vi "Analog Input.vi"() -> ()   [LabVIEW 2016]
doc: "This VI will read single point values from 4 channels of a R Series board at a specified rate."
uses:
  <vilib>/rvi/Emulation/niFpgaGetClockAttributes.vi
  <vilib>/rvi/Emulation/niFpgaSctlEmulationGetInTimedLoop.vi
  <vilib>/rvi/Emulation/niFpgaEmulationReportErrorSimple.vi
  Instance           1 27Saved   Analog Input (FPGA) .vi
  <vilib>/rvi/eio/common/nirviEmuTemplateMethod_errors.vi
  <vilib>/rvi/Emulation/niFpgaCriticalErrorInLSC.vi
  <vilib>/eio/EIONode/EIONode.xnode
panel:
  out "AI Data":T1
  in  "Loop Rate (uS)":u32=10
  # "Overview: Demonstrates the use of the analog input FPGA I/O on R Series devices.\nRequirements: LabVIEW FPGA Module, NI-RIO\nInstructions: \nRun the VI."
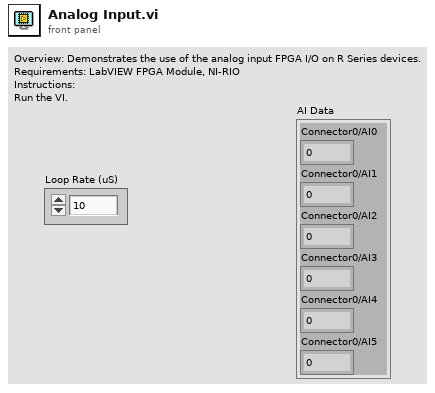
[diagram p1: front panel]
types:
  T1 = cluster{"Connector0/AI0":fxp<+/-,27,5>, "Connector0/AI1":fxp<+/-,27,5>, "Connector0/AI2":fxp<+/-,27,5>, "Connector0/AI3":fxp<+/-,27,5>, "Connector0/AI4":fxp<+/-,27,5>, "Connector0/AI5":fxp<+/-,27,5>}
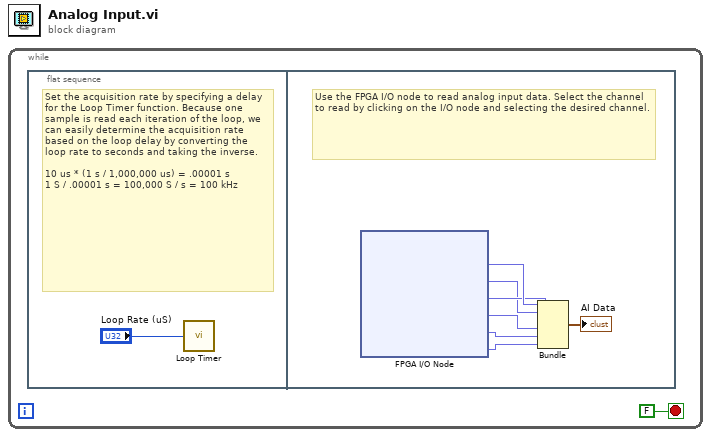
[diagram p0: block diagram]
diagram:
  n1 = while {
    stop <- FALSE ("Stop") stop-if-true
    # "Main Processing Loop"
    n2 = flat-sequence {
      frame #0 {
        # "Set the acquisition rate by specifying a delay for the Loop Timer function. Because one sample is read each iteration of the loop, we can easily determine the acquisition rate based on the loop delay by converting the loop rate to seconds and taking the inverse. \n\n10 us * (1 s / 1,000,000 us) = .00001 s\n1 S / .00001 s = 100,000 S / s = 100 kHz"
        n3 = call "Loop Timer"("Count(uSec)"="Loop Rate (uS)") -> ()  [unwired: 1 out]
      }
      frame #1 {
        # "Use the FPGA I/O node to read analog input data. Select the channel to read by clicking on the I/O node and selecting the desired channel."
        n4 = xnode "FPGA I/O Node"() -> ("Connector0/AI0"=w9:fxp<+/-,27,5>, "Connector0/AI1"=w6:fxp<+/-,27,5>, "Connector0/AI2"=w8:fxp<+/-,27,5>, "Connector0/AI3"=w7:fxp<+/-,27,5>, "Connector0/AI4"=w5:fxp<+/-,27,5>, "Connector0/AI5"=w4:fxp<+/-,27,5>)  [unwired: 7 in, 7 out]
        n5 = Bundle("Connector0/AI0"=w9, "Connector0/AI1"=w6, "Connector0/AI2"=w8, "Connector0/AI3"=w7, "Connector0/AI4"=w5, "Connector0/AI5"=w4) -> (→"AI Data":T1)  [unwired: 1 out]
      }
    }
  }
